vi "FPGA_Simuation.vi"() -> ()   [LabVIEW 2014]
uses:
  <vilib>/LabVIEW Targets/FPGA/cRIO/shared/nicrio_ModuleControls/nicrio_cRIO-9237_ExcitationVoltageRing.ctl
  <vilib>/rvi/Emulation/niFpgaGetClockAttributes.vi
  <vilib>/rvi/Emulation/niFpgaSctlEmulationGetInTimedLoop.vi
  <vilib>/rvi/Emulation/niFpgaEmulationReportErrorSimple.vi
  <vilib>/rvi/eio/common/nirviEmuTemplateMethod_errors.vi
  <vilib>/rvi/Emulation/niFpgaCriticalErrorInLSC.vi
  <vilib>/rvi/eio/common/nirviEmuTemplatePropertySet_noerrors.vi
  <vilib>/eio/EIONode/EIONode.xnode
  <vilib>/eio/EIOPropertyNode/EIOPropertyNode.xnode
  <vilib>/rvi/eio/common/nirviEmuTemplatePropertyGet_errors.vi
  <vilib>/rvi/eio/common/nirviEmuTemplatePropertyGet_noerrors.vi
  <vilib>/rvi/eio/common/nirviEmuTemplatePropertySet_errors.vi
panel:
  out "Mod1/AI4":fxp<+/-,16,5>
  out "Mod1/AI3":fxp<+/-,16,5>
  out "Mod1/AI2":fxp<+/-,16,5>
  out "Mod4/AI1":fxp<+/-,24,-4>
  out "Mod4/AI0":fxp<+/-,24,-4>
  in  "Excitation Voltage":T1 items=["2.5 Volts", "3.3 Volts", "5.0 Volts", "10.0 Volts", "External Excitation"]
  in  "Force M":bool
  out "Mod1/AI1":fxp<+/-,16,5>
  in  "Mod2/AO3":fxp<+/-,20,5>
  in  "Mod2/AO2":fxp<+/-,20,5>
  in  "Mod2/AO1":fxp<+/-,20,5>
  in  "Mod2/AO0":fxp<+/-,20,5>
  out "Mod1/AI0":fxp<+/-,16,5>
  in  "CW":bool
  in  "Width":u32 caption="Width(uSec)"
  in  "Period":u32 caption="Period(uSec)"
  in  "Move":bool
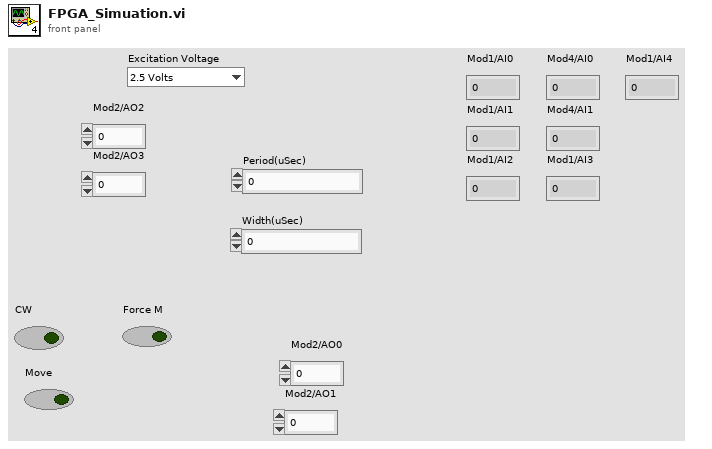
[diagram p1: front panel]
types:
  T1 = typedef "nicrio_cRIO-9237_ExcitationVoltageRing.ctl" = u8
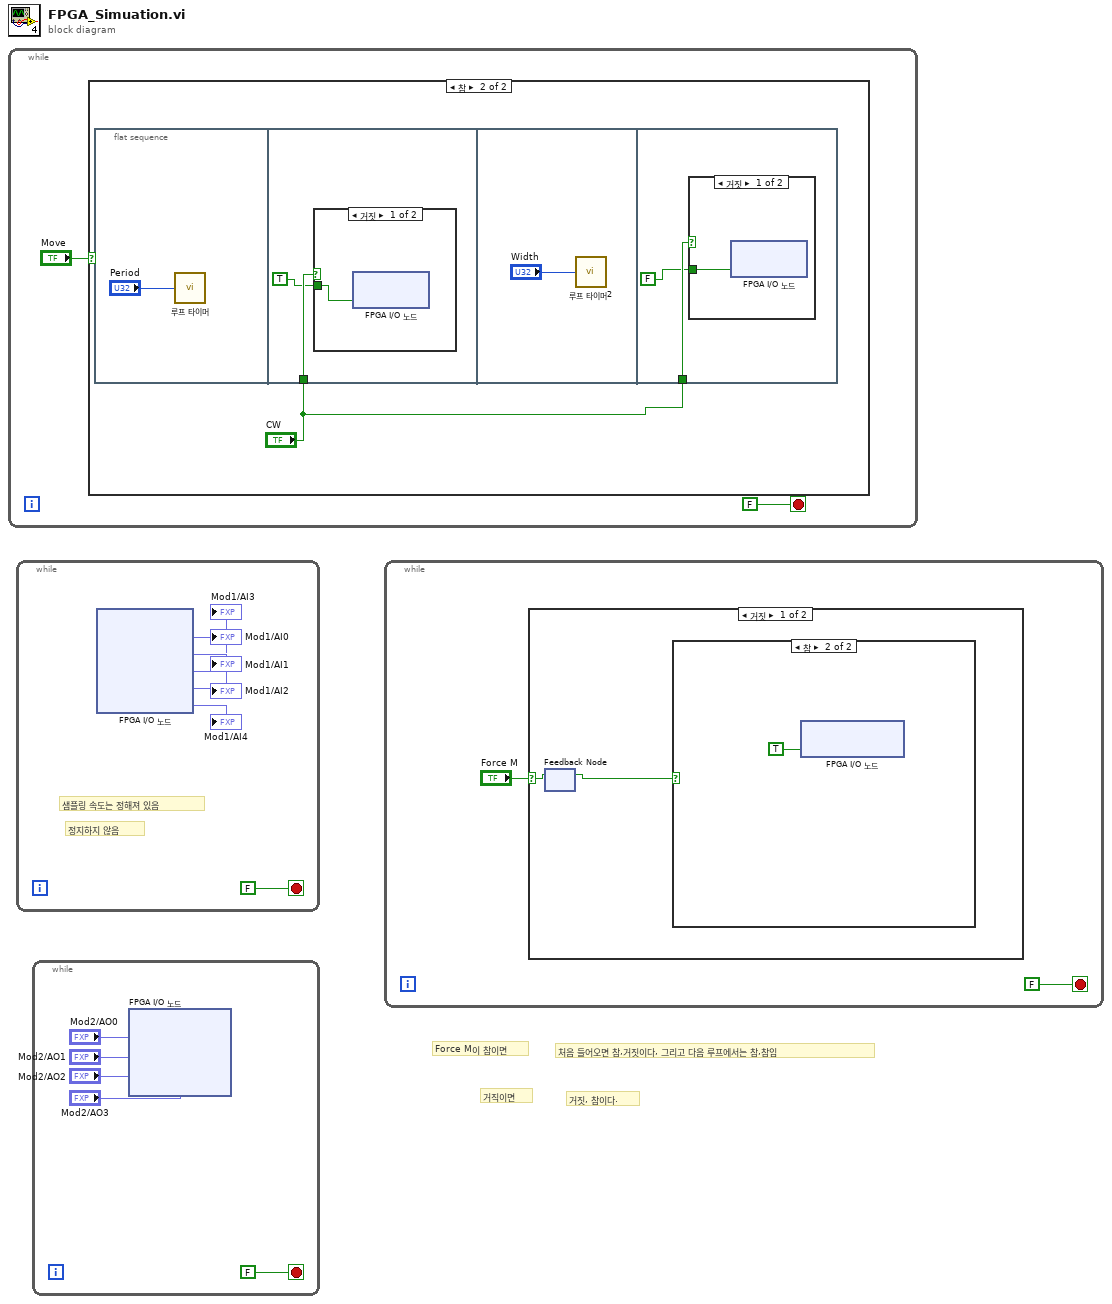
[diagram p0: block diagram]
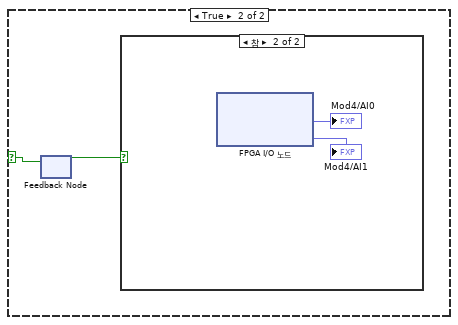
[diagram p3: hidden frame]
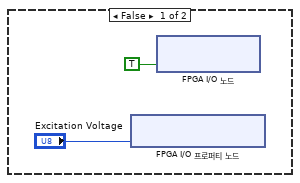
[diagram p4: hidden frame]
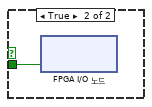
[diagram p6: hidden frame]
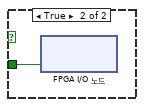
[diagram p7: hidden frame]
diagram:
  # "거짓, 참이다."
  # "거직이면"
  # "Force M이 참이면"
  # "처음 들어오면 참,거짓이다, 그리고 다음 루프에서는 참,참임"
  n1 = while {
    stop <- FALSE stop-if-true
    n2 = case shown="참" "Move" {
      frame False {
      }
      frame True {
        n3 = flat-sequence {
          tunnel: "CW" -> [w6]
          tunnel: "CW" -> [w11]
          frame #0 {
            n4 = call "루프 타이머"("Count(uSec)"="Period") -> ()  [unwired: 1 out]
          }
          frame #1 {
            n5 = case shown="거짓" w6 {
              tunnel: TRUE ("CW") -> [w7 w8]
              frame False {
                n6 = xnode "FPGA I/O 노드"("CCW"=w7) -> ()  [unwired: 1 in, 1 out]
              }
              frame True {
                n7 = xnode "FPGA I/O 노드"("CW"=w8) -> ()  [unwired: 1 in, 1 out]
              }
            }
          }
          frame #2 {
            n8 = call "루프 타이머2"("Count(uSec)"="Width") -> ()  [unwired: 1 out]
          }
          frame #3 {
            n9 = case shown="거짓" w11 {
              tunnel: FALSE ("CW") -> [w12 w13]
              frame False {
                n10 = xnode "FPGA I/O 노드"("CCW"=w12) -> ()  [unwired: 1 in, 1 out]
              }
              frame True {
                n11 = xnode "FPGA I/O 노드"("CW"=w13) -> ()  [unwired: 1 in, 1 out]
              }
            }
          }
        }
      }
    }
  }
  n12 = while {
    stop <- FALSE stop-if-true
    # "정지하지 않음"
    # "샘플링 속도는 정해져 있음"
    n13 = xnode "FPGA I/O 노드"() -> ("Mod1/AI0"=→"Mod1/AI0":fxp<+/-,16,5>, "Mod1/AI1"=→"Mod1/AI1":fxp<+/-,16,5>, "Mod1/AI2"=→"Mod1/AI2":fxp<+/-,16,5>, "Mod1/AI3"=→"Mod1/AI3":fxp<+/-,16,5>, "Mod1/AI4"=→"Mod1/AI4":fxp<+/-,16,5>)  [unwired: 5 in, 5 out]
  }
  n14 = while {
    stop <- FALSE stop-if-true
    n15 = xnode "FPGA I/O 노드"("Mod2/AO0"="Mod2/AO0", "Mod2/AO1"="Mod2/AO1", "Mod2/AO2"="Mod2/AO2", "Mod2/AO3"="Mod2/AO3") -> ()  [unwired: 4 in, 4 out]
  }
  n16 = while {
    stop <- FALSE stop-if-true
    n17 = case shown="거짓" "Force M" {
      selector: "Force M" -> [w28 w31]
      frame False {
        n18 = feedback-in #1(w28) -> ()
        n19 = feedback #1() -> (w27:bool)  [unwired: 1 in]
        n20 = case shown="참" w27 {
          frame False {
          }
          frame True {
            n21 = xnode "FPGA I/O 노드"("Mod4/Stop"=TRUE) -> ()  [unwired: 1 in, 1 out]
          }
        }
      }
      frame True {
        n22 = feedback-in #2(w31) -> ()
        n23 = feedback #2() -> (w30:bool)  [unwired: 1 in]
        n24 = case shown="참" w30 {
          frame False {
            n25 = xnode "FPGA I/O 프로퍼티 노드"("Excitation Voltage"="Excitation Voltage") -> ()  [unwired: 1 in, 1 out]
            n26 = xnode "FPGA I/O 노드"("Mod4/Start"=TRUE) -> ()  [unwired: 1 in, 1 out]
          }
          frame True {
            n27 = xnode "FPGA I/O 노드"() -> ("Mod4/AI0"=→"Mod4/AI0":fxp<+/-,24,-4>, "Mod4/AI1"=→"Mod4/AI1":fxp<+/-,24,-4>)  [unwired: 2 in, 2 out]
          }
        }
      }
    }
  }
